vi "SetPower(General).vi"(8 "Error In":errorcluster, 10 "Power":i16 min=0 max=1000, 11 "VISA resource name":refnum<visa-resource-name>) -> (0 "Error Out":errorcluster, 3 "VISA resource name out":refnum<visa-resource-name>)   [LabVIEW 2013]
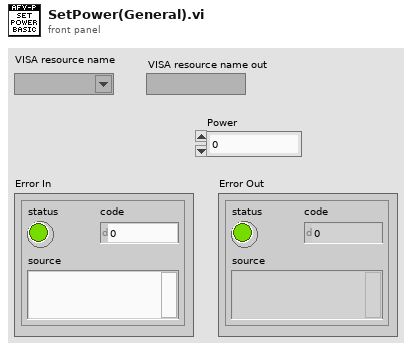
[diagram p1: front panel]
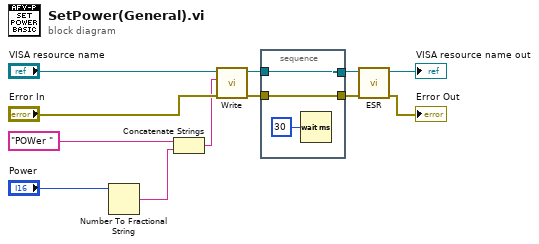
[diagram p0: block diagram]
diagram:
  n1 = Number To Fractional String(number="Power") -> (F-format string=w7:string)  [unwired: 3 in]
  n2 = Concatenate Strings("POWer " ("Write Buffer"), w7) -> (w8:string)
  n3 = call "Write.vi"("Error In"="Error In", "Write Buffer"=w8, "VISA resource name"="VISA resource name") -> ("Error Out"=w3:errorcluster, "VISA resource name out"=w4:refnum<visa-resource-name>)  [unwired: 7 in]
  n4 = stacked-sequence {
    tunnel: [w14] -> w6
    tunnel: w4 -> [w14]
    tunnel: [w13] -> w5
    tunnel: w3 -> [w13]
    frame #0 {
      n5 = Wait (ms)(milliseconds to wait=u32 30) -> ()  [unwired: 1 out]
    }
  }
  n6 = call "ESR.vi"("Error In"=w5, "VISA resource name"=w6) -> ("Error Out"=→"Error Out":errorcluster, "VISA resource name out"=→"VISA resource name out":refnum<visa-resource-name>)  [unwired: 8 in]
